vi "oa_Interpolate Tach Pulses.vi"(4 "zero delay? (F)":bool, 6 "resolution":u16(ring) items=["normal", "high"], 7 "reset? (True)":bool=TRUE, 8 "error in (no error)":errorcluster, 9 "interpolation factor":i32=4, 10 "pulse positions [s]":dbl[](array[numeric]) format="%.2f", 11 "scaled signals (EU)":waveform(dbl)[](array[waveform])) -> (0 "error out":errorcluster, 2 "interpolated pulse positions[s]":dbl[](array[numeric]) format="%.2f", 3 "dup scaled signals (EU)":waveform(dbl)[](array[waveform]), 5 "reset out":bool)   [LabVIEW 2017, in "SoundVib_Resampling.lvlib"]
doc: "Interpolates the tachometer pulses contained in <B>pulse positions [s]</B> using <B>pulse/revolution wanted</B>. Use this VI to obtain the resample time indexes before performing resampling."
uses:
  <vilib>/addons/Sound and Vibration/Order Analysis/Resample Order Tracking/SoundVib_Resampling.lvlib
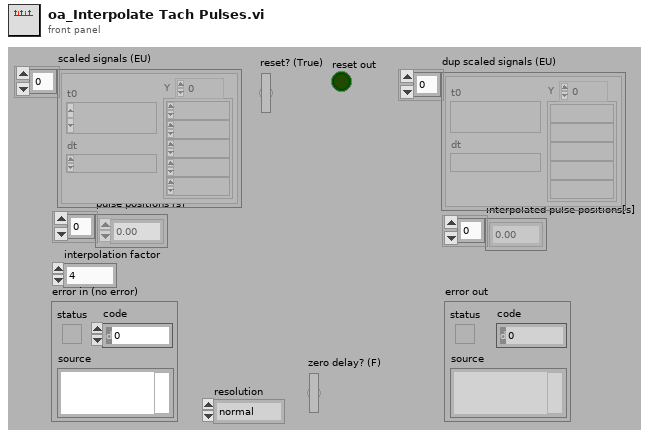
[diagram p1: front panel]
types:
  T1 = cluster{"interpolation factor":i32, "points":i32, "lag":i32}
  T2 = cluster{"interpolation factor":i32, "points":i32, "lag":i32}[]
  T3 = typedef "OAT Decimation Filter.ctl" = cluster{"coefficients":dbl[], "factor":i32}
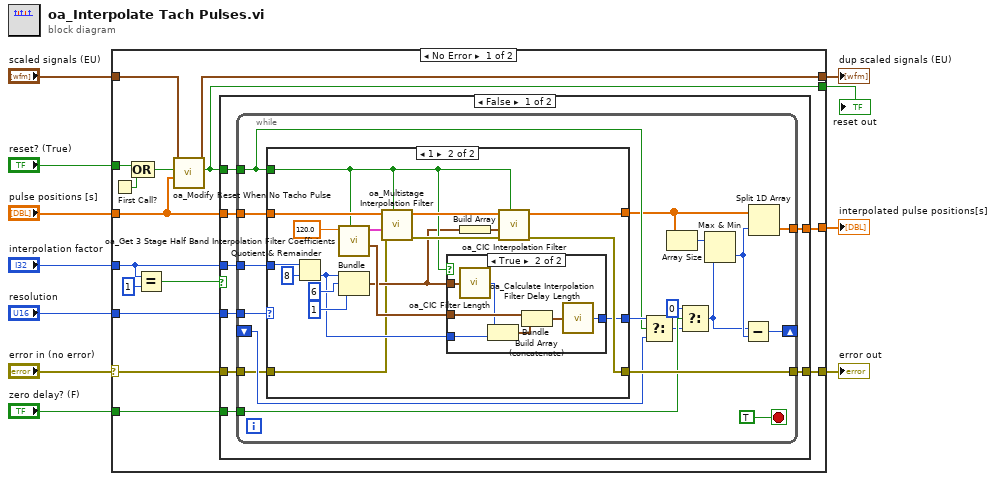
[diagram p0: block diagram]
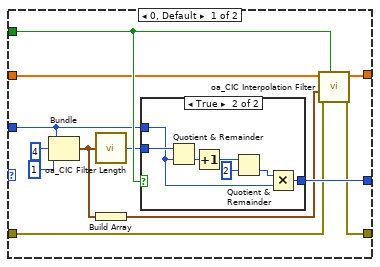
[diagram p2: hidden frame]
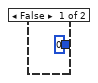
[diagram p3: hidden frame]
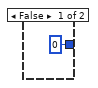
[diagram p4: hidden frame]
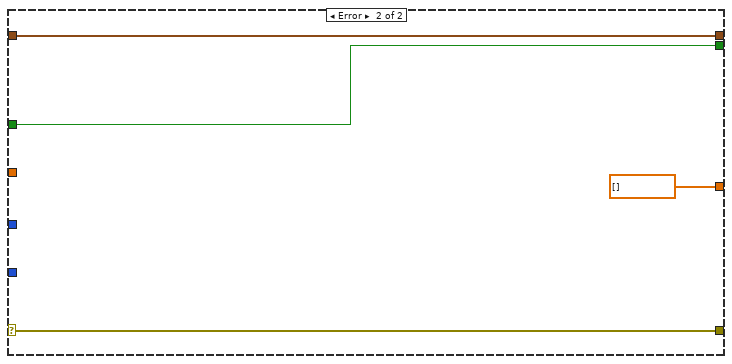
[diagram p6: hidden frame]
diagram:
  n1 = case shown="No Error" "error in (no error)" {
    selector: "error in (no error)" -> [w20 w103]
    tunnel: "pulse positions [s]" -> [w15 _]
    tunnel: "interpolation factor" -> [w23 _]
    tunnel: [w24 dbl[] [] ("Y")] -> w8
    tunnel: [w25 w103] -> w11
    tunnel: "resolution" -> [w26 _]
    tunnel: "reset? (True)" -> [w19 w101]
    tunnel: "scaled signals (EU)" -> [w17 w102]
    tunnel: [w14 w102] -> w3
    tunnel: "zero delay? (F)" -> [w13 _]
    tunnel: [w12 w101] -> w1
    frame No Error {
      n2 = First Call?() -> (First Call?: T/F=w18:bool)
      n3 = Compound Arithmetic op=OR(w19, w18) -> (w16:bool)
      n4 = Equal?(x=w23, y=1) -> (x = y?=w21:bool)
      n5 = call <vilib>:"oa_Modify Reset When No Tacho Pulse.vi"("pulse positions [s]"=w15, "reset? (True)"=w16, "scaled signals (EU)"=w17) -> ("reset out"=w12:bool, "dup scaled signals (EU)"=w14:waveform(dbl)[])  [unwired: 7 in]
      n6 = case shown="False" w21 {
        tunnel: w15 -> [w34 w100]
        tunnel: w26 -> [w33 _]
        tunnel: [w32 w99] -> w25
        tunnel: w12 -> [w31 _]
        tunnel: [w30 w100] -> w24
        tunnel: w23 -> [w29 _]
        tunnel: w20 -> [w28 w99]
        tunnel: w13 -> [w27 _]
        frame False {
          n7 = while {
            tunnel: w34 -> [w52]
            tunnel: w29 -> [w51]
            tunnel: w33 -> [w50]
            tunnel: [w49] -> w32
            tunnel: w31 -> [w43]
            tunnel: [w40] -> w30
            shift-right: [w44] -> _
            shift-left: _ -> [w46]
            tunnel: w28 -> [w39]
            tunnel: w27 -> [w38]
            stop <- TRUE stop-if-true
            n8 = case shown="1" w50 {
              tunnel: w43 -> [w61 w76]
              tunnel: w51 -> [w58 w88]
              tunnel: [w59 w80] -> w49
              tunnel: w52 -> [w54 w83]
              tunnel: [w57 w78] -> w42
              tunnel: [w64 w74] -> w47
              tunnel: w39 -> [w53 w73]
              frame 0, Default {
                n9 = Bundle("interpolation factor"=w58, "points"=4, "lag"=1) -> (w56:T1)  [unwired: 1 in]
                n10 = call <vilib>:"oa_CIC Filter Length.vi"("CIC filter settings"=w56) -> ("CIC filter length"=w55:i32)  [unwired: 14 in]
                n11 = Build Array(w56) -> (w60:T2)
                n12 = case shown="True" w61 {
                  tunnel: [0 w71] -> w64
                  tunnel: w55 -> [_ w70]
                  tunnel: w58 -> [_ w67]
                  frame False {
                  }
                  frame True {
                    n13 = Quotient & Remainder(x=w70, y=w67) -> (floor(x/y)=w69:i32)  [unwired: 1 out]
                    n14 = Increment(x=w69) -> (x+1=w68:i32)
                    n15 = Quotient & Remainder(x=w68, y=2) -> (floor(x/y)=w66:i32)  [unwired: 1 out]
                    n16 = Multiply(x=w66, y=w67) -> (x*y=w71:i32)
                  }
                }
                n17 = call <vilib>:"oa_CIC Interpolation Filter.vi"("reset? (True)"=w61, "error in (no error)"=w53, "CIC filter settings"=w60, "X"=w54) -> ("error out"=w59:errorcluster, "Y"=w57:dbl[])  [unwired: 6 in]
              }
              frame 1 {
                n18 = Quotient & Remainder(x=w88, y=8) -> (floor(x/y)=w77:i32)  [unwired: 1 out]
                n19 = call <vilib>:"oa_Get 3 Stage Half Band Interpolation Filter Coefficients.vi"("reset? (True)"=w76, "A stop [dB]"=120.0) -> ("interpolation filter info"=w85:cluster{i32, "y":i32}[], "interpolation filters"=w84:T3[])  [unwired: 8 in]
                n20 = Bundle(w77, "y"=6, "y"=1) -> (w75:cluster{i32, "y":i32, "y":i32})  [unwired: 1 in]
                n21 = call <vilib>:"oa_Multistage Interpolation Filter.vi"("reset? (True)"=w76, "error in (no error)"=w73, "interpolation filters"=w84, "x[n]"=w83) -> ("error out"=w82:errorcluster, "x[n] out"=w79:dbl[])  [unwired: 6 in]
                n22 = case shown="True" w76 {
                  tunnel: [0 w96] -> w74
                  tunnel: w85 -> [_ w95]
                  tunnel: w77 -> [_ w94]
                  tunnel: w75 -> [_ w93]
                  frame False {
                  }
                  frame True {
                    n23 = call <vilib>:"oa_CIC Filter Length.vi"("CIC filter settings"=w93) -> ("CIC filter length"=w92:i32)  [unwired: 14 in]
                    n24 = Bundle("CIC filter length"=w92, w94) -> (w98:cluster{"CIC filter length":i32, i32})  [unwired: 1 in]
                    n25 = Build Array (concatenate)(w95, w98) -> (w97:cluster{"CIC filter length":i32, "y":i32}[])
                    n26 = call <vilib>:"oa_Calculate Interpolation Filter Delay Length.vi"("filter info input"=w97) -> ("delay length"=w96:i32)
                  }
                }
                n27 = Build Array(w75) -> (w81:cluster{i32, "y":i32, "y":i32}[])
                n28 = call <vilib>:"oa_CIC Interpolation Filter.vi"("reset? (True)"=w76, "error in (no error)"=w82, "CIC filter settings"=w81, "X"=w79) -> ("error out"=w80:errorcluster, "Y"=w78:dbl[])  [unwired: 6 in]
              }
            }
            n29 = Select(t=w47, s=w43, f=w46) -> (s? t:f=w36:i32)
            n30 = Array Size(array=w42) -> (size(s)=w48:i32)
            n31 = Select(t=0 ("x"), s=w38, f=w36) -> (s? t:f=w35:i32)
            n32 = Max & Min(x=w48, y=w35) -> (min(x,y)=w41:i32)  [unwired: 1 out]
            n33 = Subtract(x=w35, y=w41) -> (x-y=w44:i32)
            n34 = Split 1D Array(array=w42, index=w41) -> (second subarray=w40:dbl[])  [unwired: 1 out]
          }
        }
        frame True {
        }
      }
    }
    frame Error {
    }
  }
  "interpolated pulse positions[s]" <- w8
  "error out" <- w11
  "dup scaled signals (EU)" <- w3
  "reset out" <- w1
